vi "Read from mpu-6050.vi"() -> (14 "Pitch":i32(knob) scale=-180.0..180.0, 15 "Roll":i32(knob) scale=-180.0..180.0, 16 "Yaw":i32(knob) scale=-180.0..180.0, 17 "A_x":dbl(slide) scale=-20.0..20.0, 18 "A_y":dbl(slide) scale=-20.0..20.0, 19 "A_z":dbl(slide) scale=-20.0..20.0)   [LabVIEW 2015]
doc: "Reads the data from the MPU-6050 inertial measurement unit and performs basic signal conditioning and interpretetion."
uses:
  MPU-6050_states_machine_state.ctl
  <vilib>/Instr/_visa.llb/VISA Configure Serial Port (Instr).vi
panel:
  out "read buffer":string
  in  "stop":bool
  out "Gx_bias":i32(knob) scale=-4.0..4.0
  # "Acceleration"
  # "Rotation"
  # "Position"
  # "x axis"
  # "y axis"
  # "z axis"
  # "Calibration"
  # "Read buffer"
  # "Gyro x-axis bias"
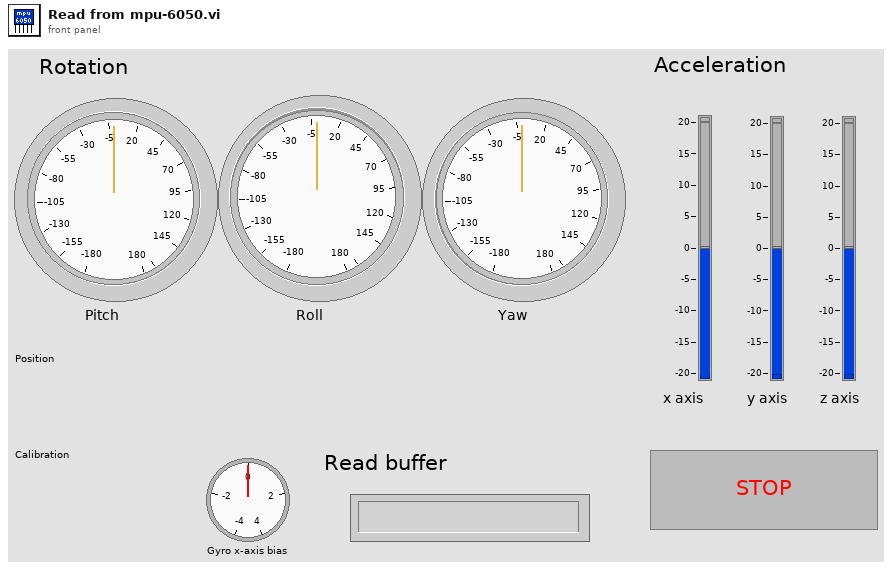
[diagram p1: front panel]
types:
  T1 = typedef "MPU-6050_states_machine_state.ctl" = enum16{"Initialize", "Calibrate", "Read", "Close", "Stop"}
  T2 = cluster{"VISA resource name":refnum<visa-resource-name>, "baud rate (9600)":u32, "Read buffer":string, "Byte count":u32, "GyroX_bias":i32, "Gravity_x":dbl, "Gravity_y":dbl, "Gravity_z":dbl, "angle_around_x":dbl, "angle_around_y":dbl, "angle_around_z":dbl}
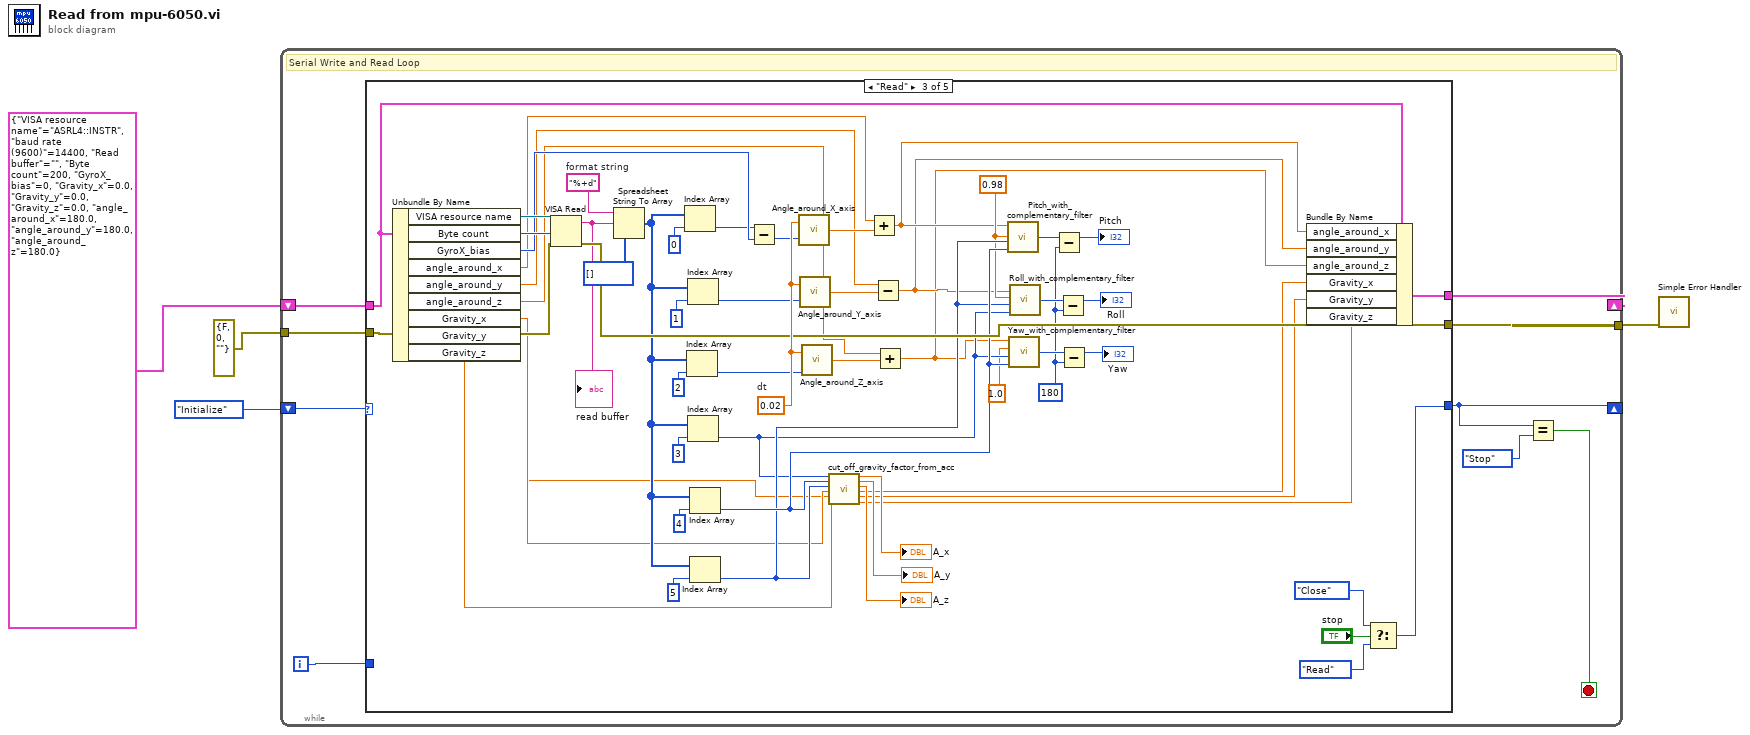
[diagram p0: block diagram]
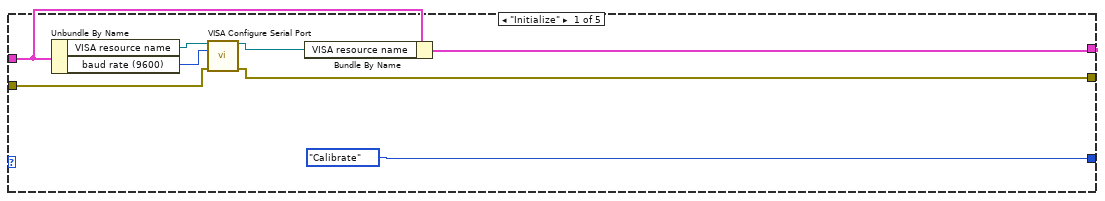
[diagram p2: hidden frame]
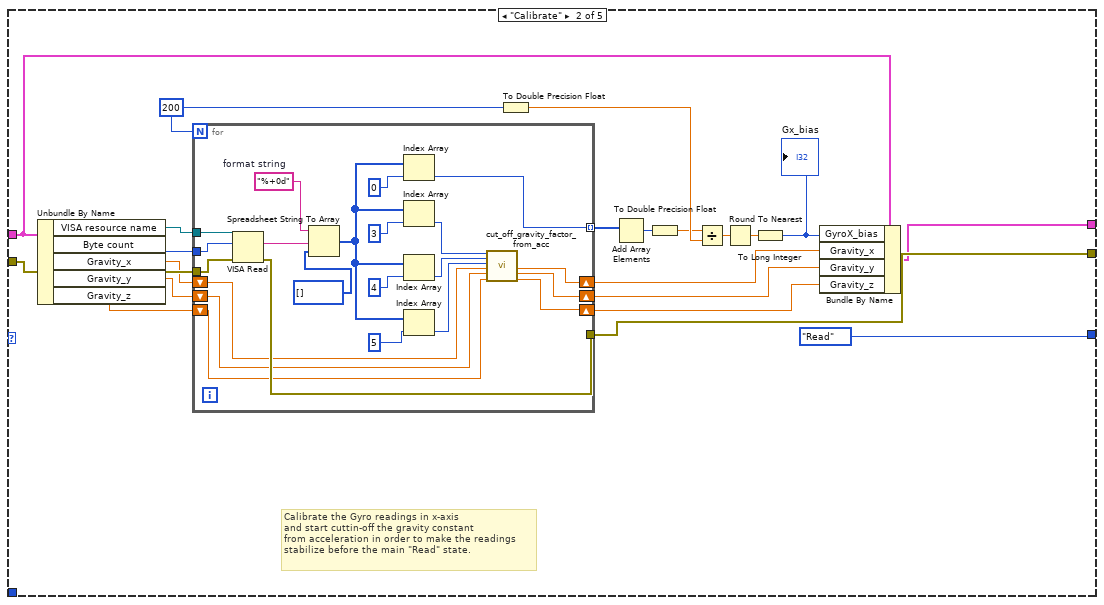
[diagram p3: hidden frame]
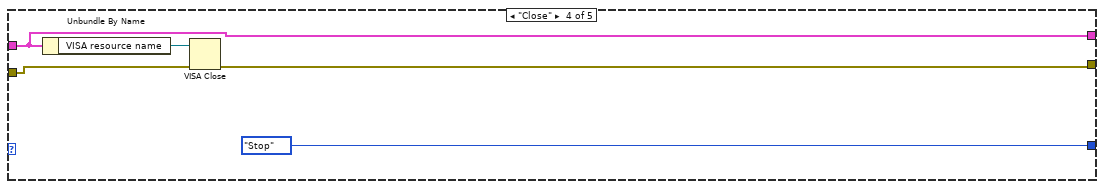
[diagram p4: hidden frame]
diagram:
  n1 = while {
    shift-right: [w11] -> _
    shift-left: T2 {"VISA resource name"="ASRL4::INSTR", "baud rate (9600)"=14400, "Read buffer"="", "Byte count"=200, "GyroX_bias"=0, "Gravity_x"=0.0, "Gravity_y"=0.0, "Gravity_z"=0.0, "angle_around_x"=180.0, "angle_around_y"=180.0, "angle_around_z"=180.0} -> [w13]
    tunnel: errorcluster {"status"=FALSE, "code"=0, "source"=""} ("error in (no error)") -> [w12]
    shift-right: [w8] -> _
    shift-left: MPU-6050_states_machine_state."Initialize" -> [w10]
    tunnel: [w9] -> w1
    i -> [w5]
    stop <- w6 stop-if-true
    # "Serial Write and Read Loop"
    n2 = case shown="\"Read\"" w10 {
      selector: w10 -> [_ _ _ _ w126]
      tunnel: w13 -> [w18 w35 w89 w123 w128]
      tunnel: w12 -> [w21 w39 w106 w124 w127]
      tunnel: [w16 w34 w88 w123 w128] -> w11
      tunnel: [MPU-6050_states_machine_state."Calibrate" MPU-6050_states_machine_state."Read" w92 MPU-6050_states_machine_state."Stop" w126] -> w8
      tunnel: [w14 w38 w105 w122 w127] -> w9
      tunnel: w5 -> [_ _ _ _ _]
      frame "Initialize" {
        n3 = Unbundle By Name(w18) -> ("VISA resource name"=w20:refnum<visa-resource-name>, "baud rate (9600)"=w19:u32)
        n4 = call-poly "VISA Configure Serial Port"("VISA resource name"=w20, "baud rate (9600)"=w19, "error in (no error)"=w21) -> ("VISA resource name out"=w17:refnum<visa-resource-name>, "error out"=w14:errorcluster)  [unwired: 11 in]
        n5 = Bundle By Name(cluster=w18, "VISA resource name"=w17) -> (w16:T2)
      }
      frame "Calibrate" {
        w37 = 200
        # "Calibrate the Gyro readings in x-axis\nand start cuttin-off the gravity constant \nfrom acceleration in order to make the readings\nstabilize before the main \"Read\" state."
        n6 = Unbundle By Name(w35) -> ("VISA resource name"=w41:refnum<visa-resource-name>, "Byte count"=w40:u32, "Gravity_x"=w27:dbl, "Gravity_y"=w26:dbl, "Gravity_z"=w25:dbl)
        n7 = for {
          N: w37 -> [_]
          tunnel: w41 -> [w64]
          tunnel: w40 -> [w63]
          tunnel: w39 -> [w62]
          tunnel: [w61] -> w38
          tunnel: [w56] -> w33 mode=indexing
          shift-right: [w45] -> w24
          shift-left: w27 -> [w48]
          shift-right: [w44] -> w23
          shift-left: w26 -> [w47]
          shift-right: [w43] -> w22
          shift-left: w25 -> [w46]
          w59 = "%+0d"  # format string
          n8 = VISA Read(VISA resource name=w64, byte count=w63, error in (no error)=w62) -> (read buffer=w58:string, error out=w61:errorcluster)  [unwired: 2 out]
          n9 = Spreadsheet String To Array(format string=w59, spreadsheet string=w58, array type (2D Dbl)=i32[] []) -> (array=w52:i32[])  [unwired: 1 in]
          n10 = Index Array "Index Array"(array=w52, index=0) -> (element=w56:i32)
          n11 = Index Array "Index Array"(array=w52, index=3) -> (element=w51:i32)
          n12 = Index Array "Index Array"(array=w52, index=4) -> (element=w50:i32)
          n13 = Index Array "Index Array"(array=w52, index=5) -> (element=w49:i32)
          n14 = call "cut_off_gravity_factor_from_acc.vi"("Ax"=w51, "Ay"=w50, "Az"=w49, "Gx_in"=w48, "Gy_in"=w47, "Gz_in"=w46) -> ("Gx_out"=w45:dbl, "Gy_out"=w44:dbl, "Gz_out"=w43:dbl)  [unwired: 8 in, 3 out]
        }
        n15 = To Double Precision Float(number=w37) -> (double precision float=w32:dbl)
        n16 = Add Array Elements(numeric array=w33) -> (sum=w36:i32)
        n17 = To Double Precision Float(number=w36) -> (double precision float=w31:dbl)
        n18 = Divide(x=w31, y=w32) -> (x/y=w30:dbl)
        n19 = Round To Nearest(number=w30) -> (nearest integer value=w29:dbl)
        n20 = To Long Integer(number=w29) -> (32bit integer=w28:i32)
        "Gx_bias" <- w28
        n21 = Bundle By Name(cluster=w35, "GyroX_bias"=w28, "Gravity_x"=w24, "Gravity_y"=w23, "Gravity_z"=w22) -> (w34:T2)
      }
      frame "Read" {
        w78 = 0.98 ("% Gyro")
        w79 = 180 ("y")
        w109 = 0.02  # dt
        w120 = "%+d"  # format string
        n22 = Unbundle By Name(w89) -> ("VISA resource name"=w108:refnum<visa-resource-name>, "Byte count"=w107:u32, "GyroX_bias"=w100:i32, "angle_around_x"=w72:dbl, "angle_around_y"=w73:dbl, "angle_around_z"=w74:dbl, "Gravity_x"=w77:dbl, "Gravity_y"=w76:dbl, "Gravity_z"=w75:dbl)
        n23 = VISA Read(VISA resource name=w108, byte count=w107, error in (no error)=w106) -> (read buffer=w96:string, error out=w105:errorcluster)  [unwired: 2 out]
        "read buffer" <- w96
        n24 = Spreadsheet String To Array(format string=w120, spreadsheet string=w96, array type (2D Dbl)=i32[] []) -> (array=w86:i32[])  [unwired: 1 in]
        n25 = Index Array "Index Array"(array=w86, index=0) -> (element=w99:i32)
        n26 = Index Array "Index Array"(array=w86, index=2) -> (element=w98:i32)
        n27 = Index Array "Index Array"(array=w86, index=1) -> (element=w97:i32)
        n28 = Index Array "Index Array"(array=w86, index=3) -> (element=w87:i32)
        n29 = Index Array "Index Array"(array=w86, index=4) -> (element=w91:i32)
        n30 = Index Array "Index Array"(array=w86, index=5) -> (element=w90:i32)
        n31 = Subtract(x=w99, y=w100) -> (x-y=w101:i32)
        n32 = call "Angle_around_X_axis.vi"("gx"=w101, "dt"=w109) -> ("Angle around the X-axis (*pitch)"=w112:dbl)
        n33 = call "Angle_around_Y_axis.vi"("gy"=w97, "dt"=w109) -> ("Angle around the Y-axis (*roll)"=w111:dbl)
        n34 = call "Angle_around_Z_axis.vi"("gz"=w98, "dt"=w109) -> ("Angle around the Z-axis (*yaw)"=w110:dbl)
        n35 = call "cut_off_gravity_factor_from_acc.vi"("Ax"=w87, "Ay"=w91, "Az"=w90, "Gx_in"=w77, "Gy_in"=w76, "Gz_in"=w75) -> ("A_x"=→"A_x":dbl, "A_y"=→"A_y":dbl, "A_z"=→"A_z":dbl, "Gx_out"=w69:dbl, "Gy_out"=w70:dbl, "Gz_out"=w71:dbl)  [unwired: 8 in]
        n36 = Add(x=w72, y=w112) -> (x+y=w68:dbl)
        n37 = Subtract(x=w73, y=w111) -> (x-y=w67:dbl)
        n38 = Add(x=w74, y=w110) -> (x+y=w66:dbl)
        n39 = call "Pitch_with_complementary_filter.vi"("ay"=w91, "az"=w90, "% Gyro"=w78, "*pitch"=w68) -> ("pitch"=w104:i32)
        n40 = call "Yaw_with_complementary_filter.vi"("ay"=w91, "ax"=w87, "% Gyro"=1.0, "*yaw"=w66) -> ("yaw"=w102:i32)
        n41 = call "Roll_with_complementary_filter.vi"("ax"=w87, "az"=w90, "% Gyro"=w78, "*roll"=w67) -> ("roll"=w103:i32)
        n42 = Subtract(x=w104, y=w79) -> (x-y=→"Pitch":i32)
        n43 = Subtract(x=w103, y=w79) -> (x-y=→"Roll":i32)
        n44 = Subtract(x=w102, y=w79) -> (x-y=→"Yaw":i32)
        n45 = Bundle By Name(cluster=w89, "angle_around_x"=w68, "angle_around_y"=w67, "angle_around_z"=w66, "Gravity_x"=w69, "Gravity_y"=w70, "Gravity_z"=w71) -> (w88:T2)
        n46 = Select(t=MPU-6050_states_machine_state."Close", s="stop", f=MPU-6050_states_machine_state."Read") -> (s? t:f=w92:T1)
      }
      frame "Close" {
        n47 = Unbundle By Name(w123) -> ("VISA resource name"=w125:refnum<visa-resource-name>)
        n48 = VISA Close(VISA resource name=w125, error in (no error)=w124) -> (error out=w122:errorcluster)
      }
      frame "Stop" {
      }
    }
    n49 = Equal?(x=w8, y=MPU-6050_states_machine_state."Stop") -> (x = y?=w6:bool)
  }
  n50 = call <vilib>:"Simple Error Handler.vi"("error in (no error)"=w1) -> ()  [unwired: 1 in, 8 out]
